vi "getMagnet.vi"(6 "Axis":T1=enum."Z", 8 "error in (no error)":errorcluster, 11 "Instrument.Cryostat in":refnum<class "Instrument.Cryostat.lvclass">) -> (0 "error out":errorcluster, 1 "Status":string, 2 "B Field (T)":dbl, 3 "Instrument.Cryostat out":refnum<class "Instrument.Cryostat.lvclass">, 4 "Finished?":bool)   [LabVIEW 2019, in "Instrument.Cryostat.lvclass"]
uses:
  Instrument.Cryostat.lvclass
  Typedefs/getMagnet--cluster.ctl
  Typedefs/Cryostat.commands--enum.ctl
  7ed934ad-8e52-49a8-b463-d59c597235b9.vi
  Typedefs/Magnet Axis--Enum.ctl
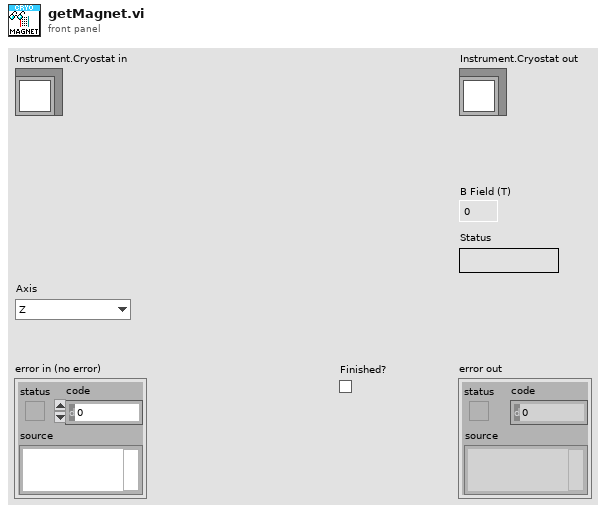
[diagram p1: front panel]
types:
  T1 = typedef "Instrument.Cryostat.lvclass/Magnet Axis--Enum.ctl" = enum16{"X", "Y", "Z"}
  T2 = typedef "Instrument.Cryostat.lvclass/Cryostat.commands--enum.ctl" = enum16{"getLN2Level", "getLHeLevel", "getMagnet", "getMagnetVector", "setMagnet", "setMagnetVector", "getAngle", "setAngle", "getTemperature", "setTemperature", "getHeater", "setHeater", "getChamber", "setChamber", "getPressure"}
  T3 = typedef "Instrument.Cryostat.lvclass/getMagnet--cluster.ctl" = cluster{"field":dbl, "status":string, "finished":bool}
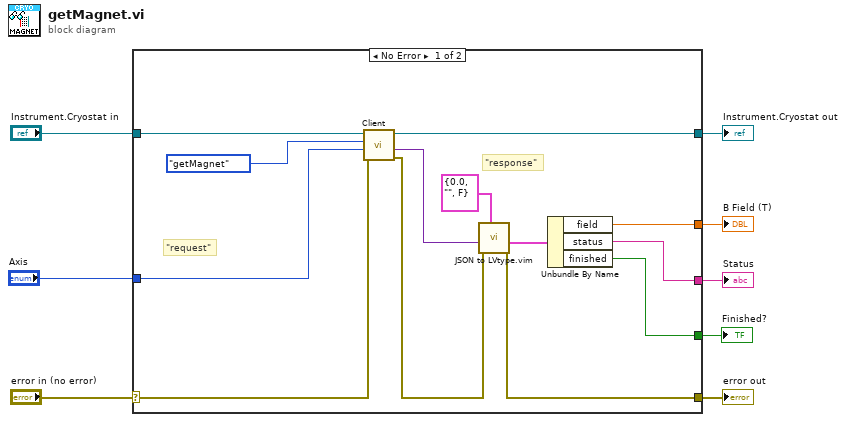
[diagram p0: block diagram]
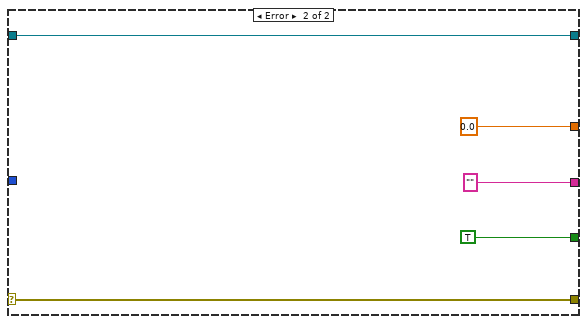
[diagram p2: hidden frame]
diagram:
  n1 = case shown="No Error" "error in (no error)" {
    selector: "error in (no error)" -> [w14 w26]
    tunnel: [w11 w26] -> w7
    tunnel: [w21 w25] -> w5
    tunnel: "Instrument.Cryostat in" -> [w16 w25]
    tunnel: "Axis" -> [w20 _]
    tunnel: [w19 0.0 ("Field (T)")] -> w3
    tunnel: [w18 "" ("Status")] -> w2
    tunnel: [w17 TRUE] -> w1
    frame No Error {
      # "\"response\""
      # "\"request\""
      n2 = call-dynamic "Client.vi"("error in (no error)"=w14, "Data in"=w20, "Command in"=Cryostat.commands--enum."getMagnet" ("commands"), "Instrument in"=w16) -> ("error out"=w12:errorcluster, "Data out"=w13:variant, "Instrument out"=w21:refnum<class "Instrument.Cryostat.lvclass">)  [unwired: 4 in, 1 out]
      n3 = call "JSON to LVtype.vim"("type"=T3 {"field"=0.0, "status"="", "finished"=FALSE} ("getMagnet"), "error in (no error)"=w12, "JSON Data in"=w13) -> ("error out"=w11:errorcluster, "Data out"=w10:T3)  [unwired: 7 in]
      n4 = Unbundle By Name(w10) -> ("field"=w19:dbl, "status"=w18:string, "finished"=w17:bool)
    }
    frame Error {
    }
  }
  "error out" <- w7
  "Instrument.Cryostat out" <- w5
  "B Field (T)" <- w3
  "Status" <- w2
  "Finished?" <- w1
